vi "CSM - MassData Data Type String.vi"(7 "error in (no error)":errorcluster, 9 "MassData Argument":string) -> (1 "error out":errorcluster, 2 "Data Type String":string, 3 "MassData Argument (dup)":string)   [LabVIEW 2017, in "CSM MassData Parameter Support.lvlib"]
doc: "Convert hex string arguments back to variant.\n\n<b>Inputs:</b>\n - <b>HEX String</b>: Hex String, which contains no invisible string following JKISM's rule\n\n<b>Outputs:</b>\n - <b>Variant</b>: Complex data in variant format."
uses:
  CSM MassData Parameter Support.lvlib
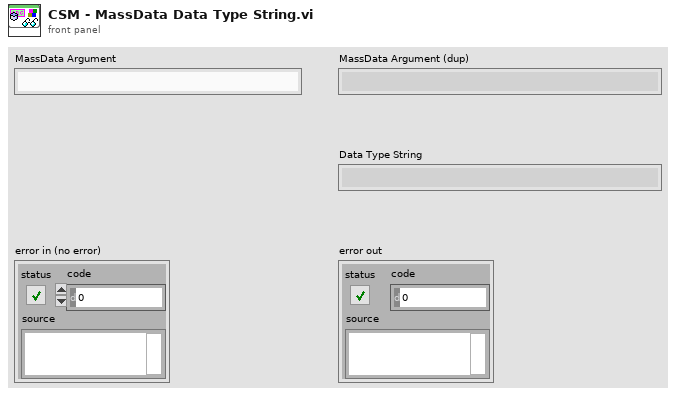
[diagram p1: front panel]
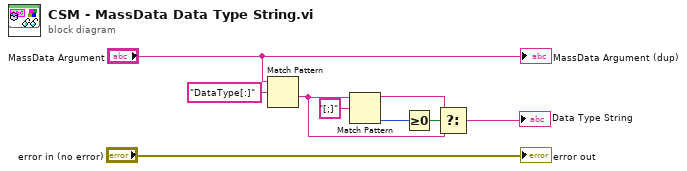
[diagram p0: block diagram]
diagram:
  n1 = Match Pattern(string="MassData Argument", regular expression="DataType[:]") -> (after substring=w2:string)  [unwired: 1 in, 3 out]
  n2 = Match Pattern(string=w2, regular expression="[;]") -> (before substring=w3:string, offset past match=w5:i32)  [unwired: 1 in, 2 out]
  n3 = Greater Or Equal To 0?(x=w5) -> (x >= 0?=w4:bool)
  n4 = Select(t=w3, s=w4, f=w2) -> (s? t:f=→"Data Type String":string)
  "MassData Argument (dup)" <- "MassData Argument"
  "error out" <- "error in (no error)"
